vi "Check Memory Objects.vi"(8 "Error In":errorcluster, 10 "Memory Object 2":T1 {"Dimension"."Width" min=1; "Dimension"."Height" min=1; "Dimension"."Depth" min=1}, 11 "Memory Object 1":T1 {"Dimension"."Width" min=1; "Dimension"."Height" min=1; "Dimension"."Depth" min=1}) -> (0 "Error Out":errorcluster)   [LabVIEW 2012, in "OpenCLV x64.lvlib"]
uses:
  OpenCLV x64.lvlib
  Controls/Memory Object.ctl
  Controls/Device ID.ctl
  Controls/Memory ID.ctl
  User Controls/Array Dimensions.ctl
  Controls/Memory Type.ctl
  Error Checking/Add Error Functional Global.vi
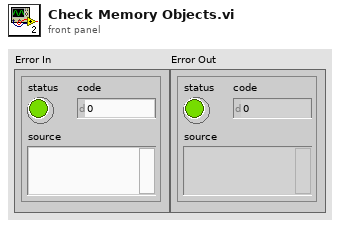
[diagram p1: front panel]
types:
  T1 = typedef "OpenCLV x64.lvlib/Memory Object.ctl" = cluster{"Device ID":T2, "Memeroy ID":T3, "Dimension":T4, "Memory Type":T5}
  T2 = typedef "OpenCLV x64.lvlib/Device ID.ctl" = u64
  T3 = typedef "OpenCLV x64.lvlib/Memory ID.ctl" = u64
  T4 = typedef "Array Dimensions.ctl" = cluster{"Depth":u64, "Height":u64, "Width":u64}
  T5 = typedef "OpenCLV x64.lvlib/Memory Type.ctl" = enum16{"32f", "u8", "i8", "u16", "i16", "u32", "i32", "64f"}
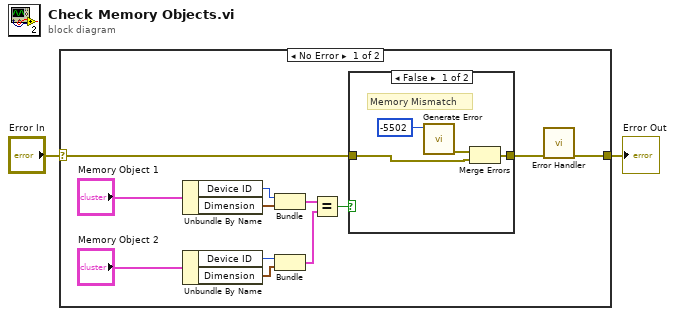
[diagram p0: block diagram]
diagram:
  n1 = case shown="No Error" "Error In" {
    selector: "Error In" -> [w5 w20]
    tunnel: [w3 w20] -> w1
    frame No Error {
      n2 = Unbundle By Name("Memory Object 1") -> ("Device ID"=w12:T2, "Dimension"=w11:T4)
      n3 = Unbundle By Name("Memory Object 2") -> ("Device ID"=w10:T2, "Dimension"=w9:T4)
      n4 = Bundle("Device ID"=w12, "Dimension"=w11) -> (w8:cluster{"Device ID":T2, "Dimension":T4})  [unwired: 1 in]
      n5 = Bundle("Device ID"=w10, "Dimension"=w9) -> (w7:cluster{"Device ID":T2, "Dimension":T4})  [unwired: 1 in]
      n6 = Equal?(x=w8, y=w7) -> (x = y?=w6:bool)
      n7 = case shown="False" w6 {
        tunnel: w5 -> [w15 w19]
        tunnel: [w17 w19] -> w4
        frame False {
          # "Memory Mismatch"
          n8 = call "Generate Error.vi"("Error"=-5502) -> ("error out"=w16:errorcluster)  [unwired: 10 in]
          n9 = Merge Errors(w16, w15) -> (w17:errorcluster)
        }
        frame True {
          # "No error"
        }
      }
      n10 = call-poly "Error Handler.vi"("Error In"=w4) -> ("Error Out"=w3:errorcluster)  [unwired: 10 in]
    }
    frame Error {
    }
  }
  "Error Out" <- w1
